vi "rszvl Query ViInt32.vi"(8 "error in (no error)":errorcluster, 9 "Command":string, 11 "VISA resource name":refnum<visa-resource-name>) -> (0 "error out":errorcluster, 2 "Value":i32, 3 "VISA resource name out":refnum<visa-resource-name>)   [LabVIEW 2014]
doc: "This VI sends the SCPI query to the instrument, reads the response and converts it to integer value."
uses:
  rszvl_rsidr_core.lvlib
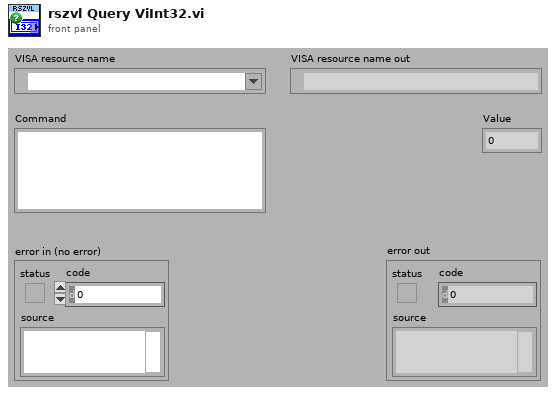
[diagram p1: front panel]
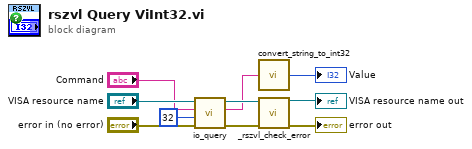
[diagram p0: block diagram]
diagram:
  n1 = call "io_query.vi"("error in"="error in (no error)", "Bytes to read (2048)"=u32 32 ("byte count"), "write buffer"="Command", "VISA resource name"="VISA resource name") -> ("error out"=w7:errorcluster, "read buffer"=w1:string, "VISA resource name out"=w4:refnum<visa-resource-name>)  [unwired: 4 in, 1 out]
  n2 = call "convert_string_to_int32.vi"("String in"=w1) -> ("int32 value out"=→"Value":i32)  [unwired: 4 in]
  n3 = call "_rszvl_check_error.vi"("VISA resource name"=w4, "error in"=w7) -> ("VISA resource name out"=→"VISA resource name out":refnum<visa-resource-name>, "error out"=→"error out":errorcluster)  [unwired: 12 in]
